vi "Clean Build Artifacts.vi"(0 "NI Build Specification in":refnum<class "SourceDist_LV.lvclass">, 11 "error in (no error)":errorcluster) -> (4 "NI Build Specification out":refnum<class "SourceDist_LV.lvclass">, 15 "error out":errorcluster)   [LabVIEW 2017, in "CL_G3_VIComponentBuilder.lvlib" / "SourceDist_LV.lvclass"]
doc: "Deletes the Directory created during build time and specified by the \"destination directory\" of the soruce distribution build spec under the info tab."
uses:
  SourceDist_LV.lvclass
  C:/builds/Component BuilderBT/SrcDist/Exports/NI Build Specification_LV/NI Build Specification_LV.lvclass
  <vilib>/AppBuilder/AB_API/common/AB_API Build Object Selector.ctl
  NI Build Specification_LV/NI Build Specification_LV.lvclass/NI Build Specification_LV.ctl
  NI Build Specification_LV/Accessors/Read TargetRef Containting Build Spec.vi
  NI Build Specification_LV/Accessors/Read Project Reference.vi
  NI Build Specification_LV/Accessors/Read Export's Build Spec Name.vi
  <vilib>/AppBuilder/AB_API/Build/NI_AB_API_Build.lvclass
  NI Build Specification_LV/NI Build Specification_LV.lvclass
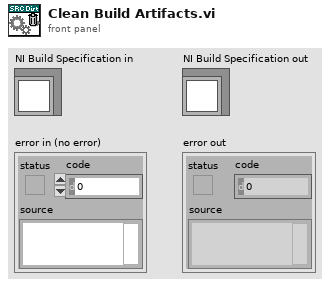
[diagram p1: front panel]
types:
  T1 = typedef "AB_API Build Object Selector.ctl" = enum16{"Source Distribution", "Deployable Source Distribution", "DLL", "EXE", "Packed Library", "Deployable Packed Library", "RT EXE", ".NET Interop Assembly"}
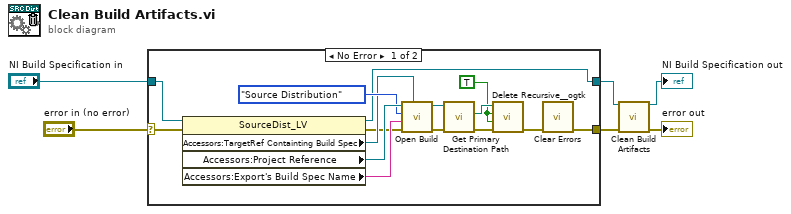
[diagram p0: block diagram]
diagram:
  n1 = case shown="No Error" "error in (no error)" {
    selector: "error in (no error)" -> [w11 w22]
    tunnel: "NI Build Specification in" -> [w10 w23]
    tunnel: [w7 w22] -> w2
    tunnel: [w8 w23] -> w1
    frame No Error {
      w13 = TRUE ("Ignore Read-Only? (FALSE)")
      n2 = property class="SourceDist_LV"(reference=w10, error in=w11) -> (reference out=w8:refnum<class "SourceDist_LV.lvclass">, error out=w16:errorcluster, "Accessors:TargetRef Containting Build Spec"=w18:refnum<vi>, "Accessors:Project Reference"=w21:refnum<vi>, "Accessors:Export's Build Spec Name"=w17:string)
      n3 = call <vilib>:"Open Build.vi"("TargetItem Refnum"=w18, "error in (no error)"=w16, "Build specification name"=w17, "Build object selector"=AB_API_Build_Object_Selector."Source Distribution", "Project Refnum"=w21) -> ("error out"=w15:errorcluster, "NI_AB_API_Build out"=w19:refnum<class "NI_AB_API_Build.lvclass">)  [unwired: 5 in]
      n4 = call-dynamic "Get Primary Destination Path.vi"("error in (no error)"=w15, "NI_AB_API_Build in"=w19) -> ("error out"=w12:errorcluster, "Primary destination path"=w14:path)  [unwired: 7 in, 1 out]
      n5 = call <userlib>:"Delete Recursive__ogtk.vi"("error in (no error)"=w12, "Ignore Read-Only? (FALSE)"=w13, "Recursive? (FALSE)"=w13, "Path"=w14) -> ("error out"=w9:errorcluster)  [unwired: 6 in, 1 out]
      n6 = call <vilib>:"Clear Errors.vi"("error in (no error)"=w9) -> ("error out"=w7:errorcluster)  [unwired: 5 in, 1 out]
    }
    frame Error {
    }
  }
  n7 = call-parent "Clean Build Artifacts.vi"("NI Build Specification in"=w1, "error in (no error)"=w2) -> ("NI Build Specification out"=→"NI Build Specification out":refnum<class "SourceDist_LV.lvclass">, "error out"=→"error out":errorcluster)  [unwired: 12 in]
